vi "Get Possition.vi"(8 "error in (no error)":errorcluster, 11 "Motor in":refnum<class "Motor.lvclass">) -> (0 "error out":errorcluster, 2 "Revolutions":dbl, 3 "Motor out":refnum<class "Motor.lvclass">)   [LabVIEW 2019, in "Motor.lvclass"]
uses:
  Motor.lvclass
  Motor.lvclass/Motor.ctl
  Motor Serial class/Serial.lvclass
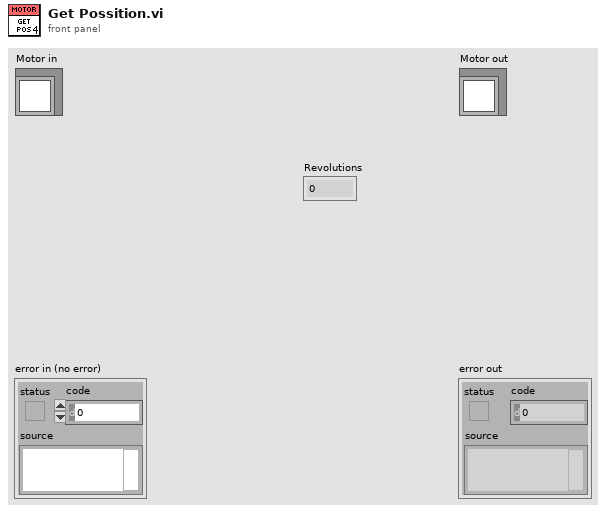
[diagram p1: front panel]
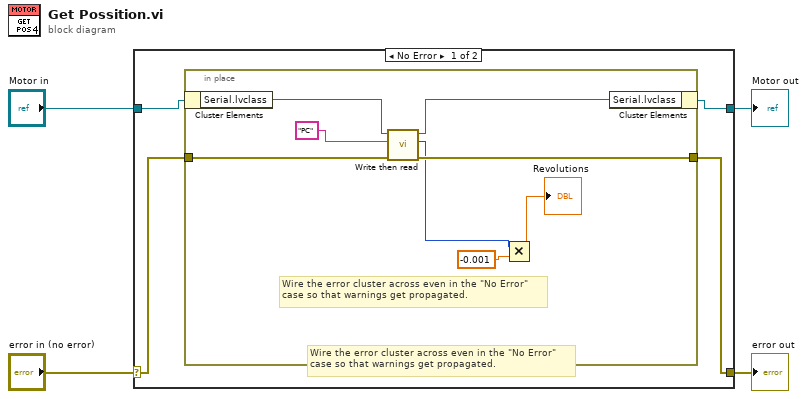
[diagram p0: block diagram]
diagram:
  n1 = case shown="No Error" "error in (no error)" {
    selector: "error in (no error)" -> [w6 w18]
    tunnel: [w5 w18] -> w3
    tunnel: [w7 w17] -> w1
    tunnel: "Motor in" -> [w8 w17]
    frame No Error {
      # "Wire the error cluster across even in the \"No Error\"\ncase so that warnings get propagated."
      n2 = in-place {
        in-place-border: w6 -> [w14]
        in-place-border: [w13] -> w5
        # "Wire the error cluster across even in the \"No Error\"\ncase so that warnings get propagated."
        n3 = in-place-cluster #1(w8) -> ("Serial.lvclass"=w16:refnum<class "Serial.lvclass">)
        n4 = call "Write then read.vi"("error in (no error)"=w14, "TX Data"="PC" ("string"), "Motor_Serial in"=w16) -> ("error out"=w13:errorcluster, "RX Data"=w9:i32, "Motor_Serial out"=w15:refnum<class "Serial.lvclass">)  [unwired: 5 in]
        n5 = Multiply(x=w9, y=-0.001) -> (x*y=→"Revolutions":dbl)
        n6 = in-place-cluster #1("Serial.lvclass"=w15) -> (w7:refnum<class "Motor.lvclass">)
      }
    }
    frame Error {
    }
  }
  "error out" <- w3
  "Motor out" <- w1
